vi "circuits-gound.vi"(1 "L3":dbl=0.1, 4 "L2":dbl=0.1, 5 "GetPOS Y":refnum<vi>, 6 "L1":dbl=0.1, 7 "GetPOS X":refnum<vi>, 8 "Device in Y":refnum<k24>, 11 "Device in X":refnum<k24>) -> (0 "Device out Y":refnum<k24>, 3 "Device out X":refnum<k24>)   [LabVIEW 2014]
doc: "André Romero - 2019\nandretec@ifsc.usp.br"
uses:
  C:/user-Lab/AndreTec/GITs/andretec/Thorlabs-Vector-Move/kinesisTec/Kinesis/Thorlabs.MotionControl.TCube.DCServoCLI.dll
  kinesisTec/Kinesis/Thorlabs.MotionControl.TCube.DCServoCLI.dll
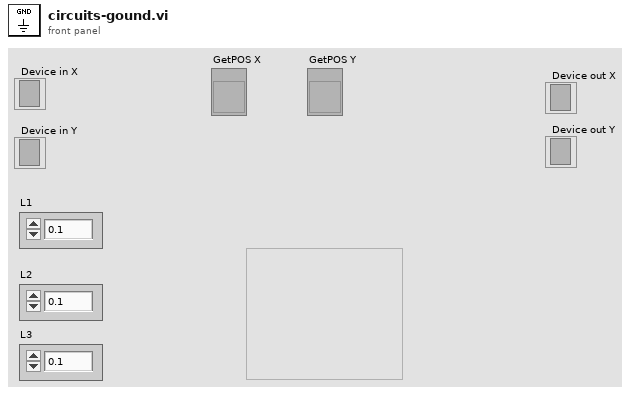
[diagram p1: front panel]
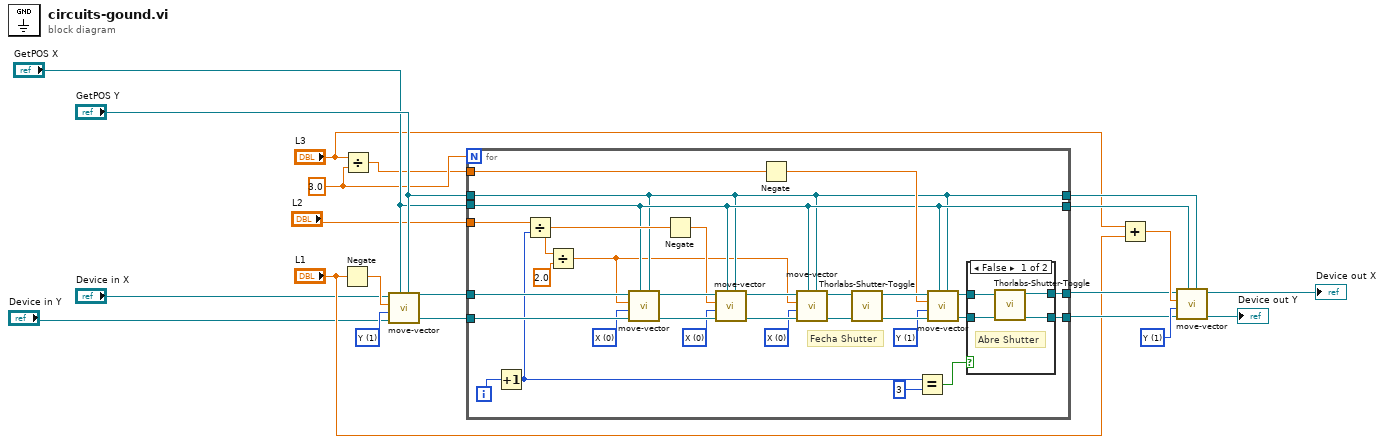
[diagram p0: block diagram]
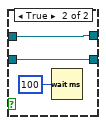
[diagram p2: hidden frame]
diagram:
  w15 = u16 1 items=["X", "Y"] ("X-Y")
  w7 = 3.0 ("y")
  w3 = u16 1 items=["X", "Y"] ("X-Y")
  n1 = Negate(x="L1") -> (-x=w8:dbl)
  n2 = Divide(x="L3", y=w7) -> (x/y=w6:dbl)
  n3 = call "move-vector.vi"("GetPOS Y"="GetPOS Y", "GetPOS X"="GetPOS X", "Device in Y"="Device in Y", "X-Y"=w3, "Distance"=w8, "Device in X"="Device in X") -> ("Device out Y"=w4:refnum<k24>, "Device out X"=w5:refnum<k24>)  [unwired: 4 in]
  n4 = for {
    N: w7 -> [_]
    tunnel: w4 -> [w52]
    tunnel: w5 -> [w51]
    tunnel: w6 -> [w37]
    tunnel: [w31] -> w13
    tunnel: [w30] -> w14
    tunnel: [w24] -> w16
    tunnel: [w23] -> w17
    tunnel: "L2" -> [w25]
    tunnel: "GetPOS X" -> [w24]
    tunnel: "GetPOS Y" -> [w23]
    i -> [w35]
    w36 = u16 1 items=["X", "Y"] ("X-Y")
    w42 = u16 0 items=["X", "Y"] ("X-Y")
    w45 = u16 0 items=["X", "Y"] ("X-Y")
    w50 = u16 0 items=["X", "Y"] ("X-Y")
    # "Fecha Shutter"
    n5 = Increment(x=w35) -> (x+1=w27:i32)
    n6 = Divide(x=w25, y=w27) -> (x/y=w32:dbl)
    n7 = Divide(x=w32, y=2.0 ("x")) -> (x/y=w22:dbl)
    n8 = call "move-vector.vi"("GetPOS Y"=w23, "GetPOS X"=w24, "Device in Y"=w52, "X-Y"=w50, "Distance"=w22, "Device in X"=w51) -> ("Device out Y"=w47:refnum<k24>, "Device out X"=w48:refnum<k24>)  [unwired: 4 in]
    n9 = Negate(x=w32) -> (-x=w46:dbl)
    n10 = call "move-vector.vi"("GetPOS Y"=w23, "GetPOS X"=w24, "Device in Y"=w47, "X-Y"=w45, "Distance"=w46, "Device in X"=w48) -> ("Device out Y"=w43:refnum<k24>, "Device out X"=w44:refnum<k24>)  [unwired: 4 in]
    n11 = Negate(x=w37) -> (-x=w29:dbl)
    n12 = call "move-vector.vi"("GetPOS Y"=w23, "GetPOS X"=w24, "Device in Y"=w43, "X-Y"=w42, "Distance"=w22, "Device in X"=w44) -> ("Device out Y"=w40:refnum<k24>, "Device out X"=w41:refnum<k24>)  [unwired: 4 in]
    n13 = call "Thorlabs-Shutter-Toggle.vi"("Device in Y"=w40, "Device in X"=w41) -> ("Device out Y"=w38:refnum<k24>, "Device out X"=w39:refnum<k24>)  [unwired: 8 in]
    n14 = Equal?(x=w27, y=3) -> (x = y?=w28:bool)
    n15 = call "move-vector.vi"("GetPOS Y"=w23, "GetPOS X"=w24, "Device in Y"=w38, "X-Y"=w36, "Distance"=w29, "Device in X"=w39) -> ("Device out Y"=w33:refnum<k24>, "Device out X"=w34:refnum<k24>)  [unwired: 4 in]
    n16 = case shown="False" w28 {
      tunnel: w34 -> [w56 w59]
      tunnel: w33 -> [w55 w58]
      tunnel: [w54 w59] -> w31
      tunnel: [w53 w58] -> w30
      frame False {
        # "Abre Shutter"
        n17 = call "Thorlabs-Shutter-Toggle.vi"("Device in Y"=w55, "Device in X"=w56) -> ("Device out Y"=w53:refnum<k24>, "Device out X"=w54:refnum<k24>)  [unwired: 8 in]
      }
      frame True {
        n18 = Wait (ms)(milliseconds to wait=u32 100) -> ()  [unwired: 1 out]
      }
    }
  }
  n19 = Add(x="L3", y="L1") -> (x+y=w18:dbl)
  n20 = call "move-vector.vi"("GetPOS Y"=w17, "GetPOS X"=w16, "Device in Y"=w14, "X-Y"=w15, "Distance"=w18, "Device in X"=w13) -> ("Device out Y"=→"Device out Y":refnum<k24>, "Device out X"=→"Device out X":refnum<k24>)  [unwired: 4 in]
